vi "Report Core.vi"(8 "error in":errorcluster, 9 "Received":path, 10 "Approved":path, 11 "Report Nothing in":refnum<class "Report With Native Compare Tool.lvclass">) -> (0 "error out":errorcluster, 2 "Worked?":bool, 3 "Report Nothing out":refnum<class "Report With Native Compare Tool.lvclass">)   [LabVIEW 2020, in "Approval Tests.lvlib" / "Report With Native Compare Tool.lvclass"]
uses:
  Report With Native Compare Tool.lvclass
  Report With Native Compare Tool.lvclass/Report With Native Compare Tool.ctl
  Diff View.vi
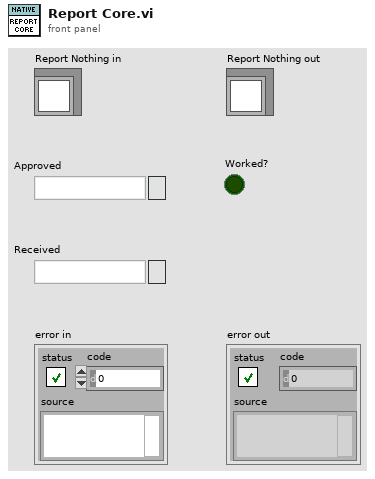
[diagram p1: front panel]
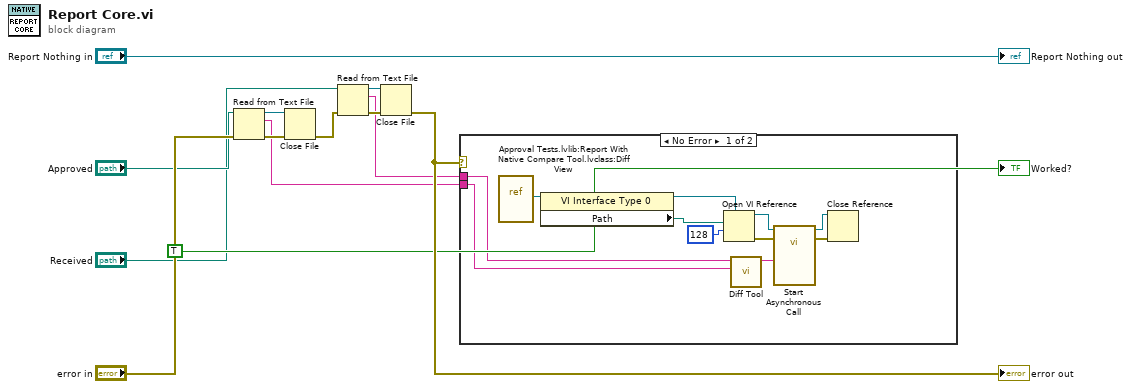
[diagram p0: block diagram]
diagram:
  n1 = Read from Text File(file (use dialog)="Approved", error in="error in") -> (refnum out=w3:refnum<file>, text=w1:string, error out=w13:errorcluster)  [unwired: 2 in, 1 out]
  n2 = Close File(refnum=w3, error in=w13) -> (error out=w12:errorcluster)  [unwired: 1 out]
  n3 = Read from Text File(file (use dialog)="Received", error in=w12) -> (refnum out=w4:refnum<file>, text=w2:string, error out=w10:errorcluster)  [unwired: 2 in, 1 out]
  n4 = Close File(refnum=w4, error in=w10) -> (error out=w9:errorcluster)  [unwired: 1 out]
  "error out" <- w9
  n5 = case shown="No Error" w9 {
    tunnel: w2 -> [w22 _]
    tunnel: w1 -> [w21 _]
    frame No Error {
      n6 = vi-ref "Approval Tests.lvlib:Report With Native Compare Tool.lvclass:Diff View.vi"() -> (w20:refnum<vi>)
      n7 = property class="VI Interface Type 0"(reference=w20) -> (reference out=w17:refnum<vi>, "Path"=w19:path)  [unwired: 1 in, 1 out]
      n8 = Open VI Reference(type specifier VI Refnum (for type only)=w17, vi path=w19, options=128) -> (vi reference=w15:refnum<vi>, error out=w24:errorcluster)  [unwired: 3 in]
      n9 = call "Diff Tool.vi"("Reference"=w21, "Target"=w22) -> ("Result"=w14:string)  [unwired: 8 in, 1 out]
      n10 = call-by-ref "Start Asynchronous Call"(reference=w15, error in=w24, "Diffed Text"=w14) -> (reference out=w16:refnum<vi>, error out=w23:errorcluster)  [unwired: 11 in]
      n11 = Close Reference(reference=w16, error in (no error)=w23) -> ()  [unwired: 1 out]
    }
    frame Error {
    }
  }
  "Report Nothing out" <- "Report Nothing in"
  "Worked?" <- TRUE ("Reporter Was Launched?")
